vi "MathBuckPr1.vi"() -> ()   [LabVIEW 2015]
uses:
  <vilib>/Simulation/Scripting/Companion Diagram/SimConfigNode/SimParams.ctl
  <vilib>/Simulation/Scripting/Companion Diagram/SimConfigNode/_simSolvers.ctl
  <vilib>/Simulation/Implementation/Shared/SIMSCR Execution Mode.ctl
  <vilib>/Simulation/Param Hierarchy/Typedefs/SIMPH Param Control Actions.ctl
  <vilib>/Simulation/Implementation/Shared/NILVSim_ParamChanged.vi
  <vilib>/Simulation/Implementation/Shared/NILVSIM_BeginStep.vi
  <vilib>/Simulation/Implementation/Shared/NILVSim_Manager.vi
  <vilib>/Utility/error.llb/Clear Errors.vi
  <vilib>/Simulation/Implementation/Shared/NILVSim_FinalizeModel.vi
  <vilib>/imath/engines/lvmath2/RunTimeEngine/Managers/WorkSpace/UID Generator.vi
  <vilib>/imath/engines/lvmath/Plug In/Control Design/BuiltInFunctions/tf/NIMS_CD_tf(STR,Ts).vi
  <vilib>/imathl/engines/lvmath/Functions/Error Handling/Create Error.vi
  <vilib>/imath/engines/lvmath/Plug In/Control Design/BuiltInFunctions/multmx/NIMS_CD_multmx(TF,K).vi
  <vilib>/imath/engines/lvmath/Plug In/Control Design/BuiltInFunctions/powermx/NIMS_CD_powermx(TF,N).vi
  <vilib>/imath/engines/lvmath/Plug In/Control Design/BuiltInFunctions/plus/NIMS_CD_plus(TF,TF).vi
  <vilib>/imath/engines/lvmath/Plug In/Control Design/BuiltInFunctions/plus/NIMS_CD_plus(TF,K).vi
  <vilib>/imath/engines/lvmath/Plug In/Control Design/BuiltInFunctions/multmx/NIMS_CD_multmx(K,TF).vi
  <vilib>/imath/engines/lvmath/Functions/Error Handling/MergeErrorsWrapper.vi
  <vilib>/imath/engines/lvmath/Plug In/Control Design/BuiltInFunctions/plus/NIMS_CD_plus(K,TF).vi
  <vilib>/imath/engines/lvmath/Plug In/Control Design/BuiltInFunctions/rightdivmx/NIMS_CD_rightdivmx(TF,TF).vi
  <vilib>/imath/engines/lvmath/Plug In/Control Design/BuiltInFunctions/rightdivmx/NIMS_CD_rightdivmx(TF,K).vi
  <vilib>/imath/engines/lvmath/Plug In/Control Design/BuiltInFunctions/step/NIMS_CD_[Y,T]=step(TF,[Tinfo]).vi
  <vilib>/imath/engines/lvmath/Plug In/Control Design/BuiltInFunctionSupport/CD_timePlotData(TF).vi
  <vilib>/imath/engines/lvmath/Plug In/Control Design/BuiltInFunctionSupport/Utility_Functions/Plot_Utility/cdmc textMathPlot.vi
  <vilib>/imath/engines/lvmath2/RunTimeEngine/Managers/SymbolTable/Clear UID.vi
  <vilib>/imath/engines/lvmath2/RunTimeEngine/NodeEndStatement/NIMS_NodeEndStatement_Output.vi
  <instcachedir>/0/NIMS_NodeEndStatement_Output_53EC0D466D134D7ABD903AC30B43404B.lvgen/NIMS_NodeEndStatement_Output_53EC0D466D134D7ABD903AC30B43404B_001.vi
  <instcachedir>/0/NIMS_NodeEndStatement_Output_53EC0D466D134D7ABD903AC30B43404B.lvgen/NIMS_NodeEndStatement_Output_53EC0D466D134D7ABD903AC30B43404B_002.vi
  <vilib>/imath/engines/lvmath2/RunTimeEngine/ErrorHandling/NIMS_Finalize Error.vi
  <vilib>/Analysis/Matrix/Numeric/Conversions/Matrix To Array - RM.vi
  <vilib>/Simulation/Implementation/Shared/SIM Unbundle Sim Info.vi
  <vilib>/Simulation/Implementation/Shared/NILVSim_Initialize.vi
  <vilib>/Simulation/Utility/Implementation/NILVSim Get Time and IsAcceptedStep.vi
  <vilib>/Simulation/Implementation/Shared/SIMSH Read Queue.vi
  <vilib>/Simulation/Implementation/Shared/NILVSim_GetModelError.vi
  <vilib>/Simulation/Implementation/Shared/SIM Bundle Sim Info.vi
  <vilib>/Simulation/Scripting/Companion Diagram/SimConfigNode/SimDog.xnode
  <vilib>/Analysis/Matrix/NI_Matrix.lvlib
  <vilib>/Simulation/Implementation/Shared/NI_SIM_Implementation.lvlib
  <vilib>/imath/engines/lvmath2/RunTimeEngine/Managers/SymbolTable/NIMS_WorkSpace.lvlib
panel:
  out "DeltaIL":dbl
  out "P":dbl
  out "Io":dbl
  out "Vo 2":dbl
  in  "error in":errorcluster
  out "Vo":dbl[](graph)
  out "IL":dbl[](graph)
  in  "r":dbl
  in  "D":dbl
  in  "F":dbl
  in  "R":dbl
  in  "C":dbl
  in  "L":dbl
  in  "Vin":dbl
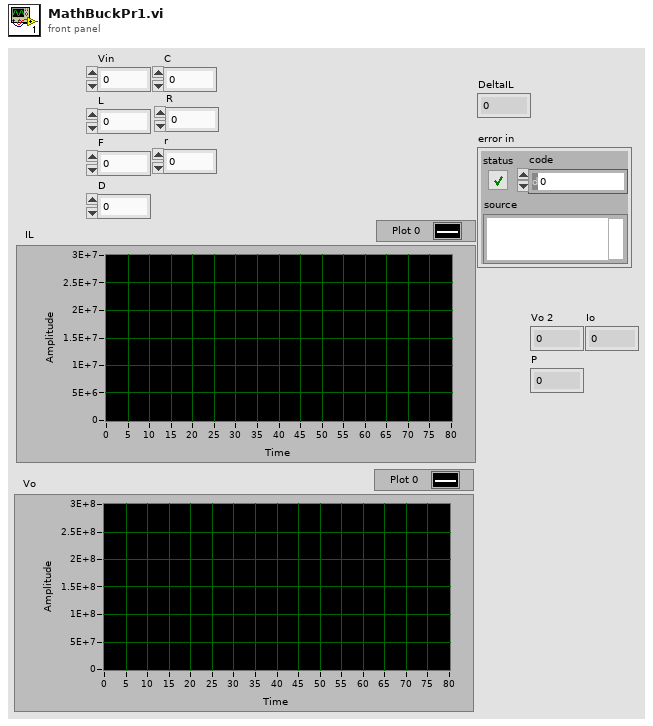
[diagram p1: front panel]
types:
  T1 = cluster{"[0]":i32, "[1]":i32, "[2]":i32, "[3]":i32, "[4]":i32, "[5]":i32, "[6]":i32, "[7]":i32, "[8]":i32}
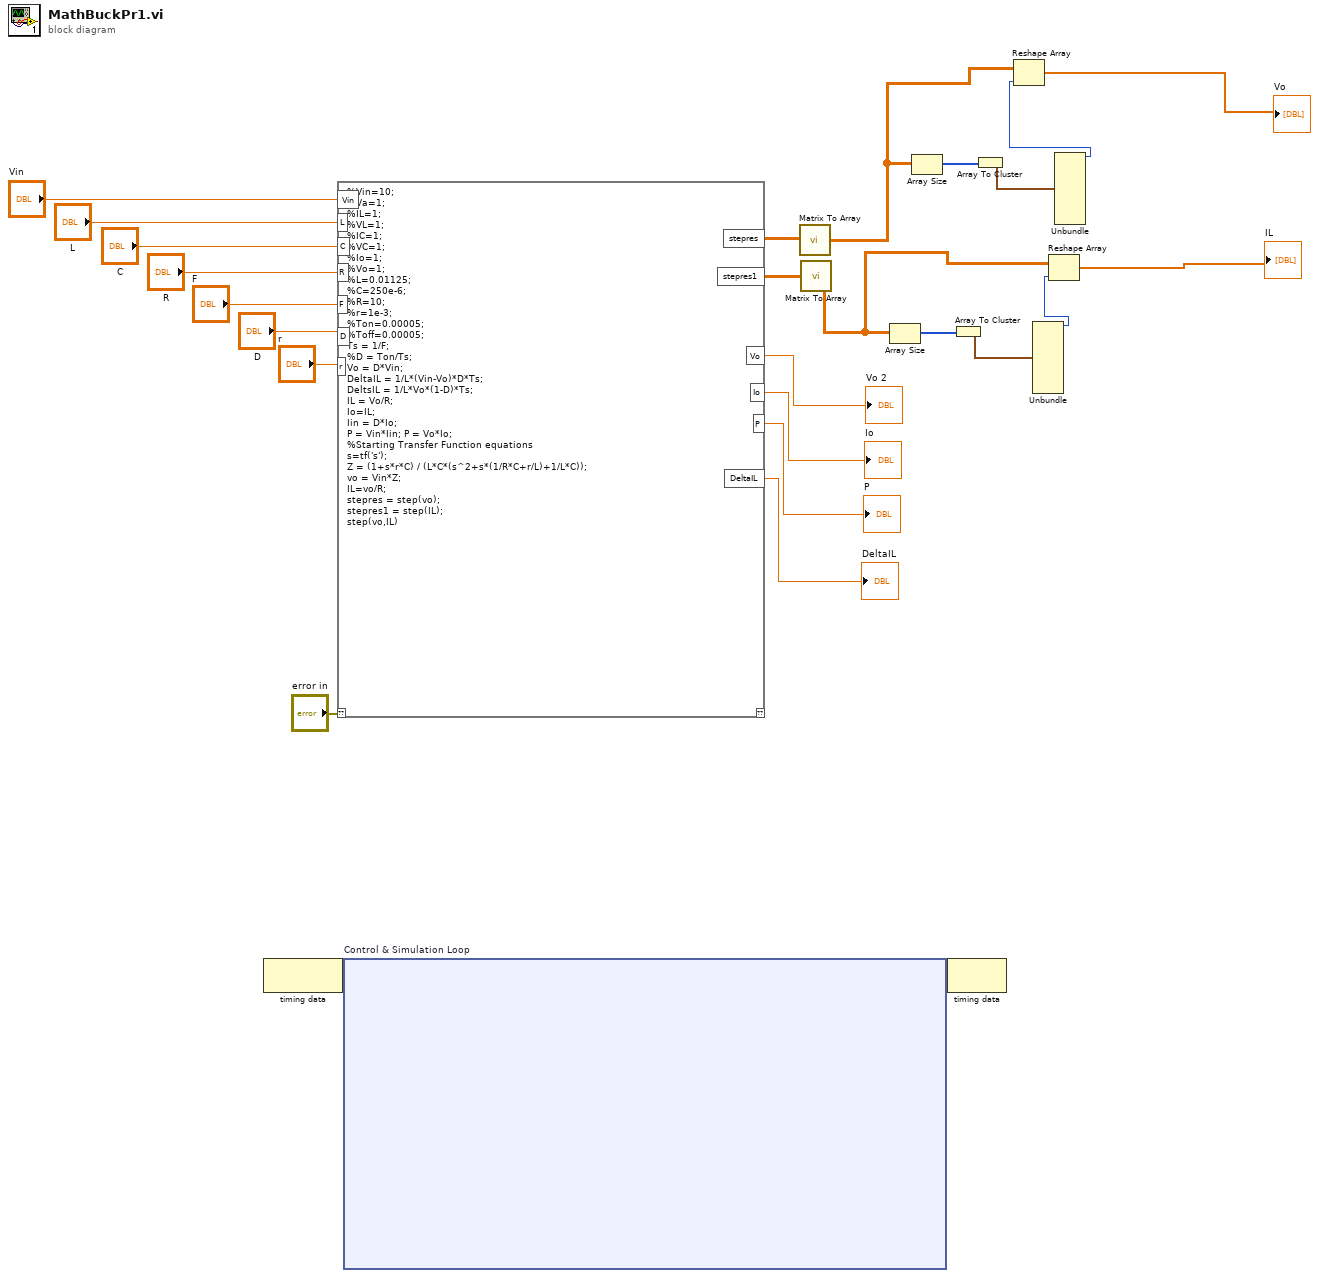
[diagram p0: block diagram]
diagram:
  n1 = node-c288() -> (w2:variant)  [unwired: 1 in]
  n2 = mathscript code="%Vin=10;\n%Va=1;\n%IL=1;\n%VL=1;\n%IC=1;\n%VC=1;\n%Io=1;\n%Vo=1;\n%L=0.01125;\n%C=250e-6;\n%R=10;\n%r=1e-3;\n%Ton=0.00005;\n%Toff=0.00005;\nTs = 1/F;\n%D = Ton/Ts;\nVo = D*Vin;\nDeltaIL = 1/L*(Vin-Vo)*D*Ts;\nDeltsIL = 1/L*Vo*(1-D)*Ts;\nIL = Vo/R;\nIo=IL;\nIin = D*Io;\nP = Vin*Iin; P = Vo*Io;\n%Starting Transfer Function equations\ns=tf('s');\nZ = (1+s*r*C) / (L*C*(s^2+s*(1/R*C+r/L)+1/L*C));\nvo = Vin*Z;\nIL=vo/R;\nstepres = step(vo);\nstepres1 = step(IL);\nstep(vo,IL)"("??"="error in", "Vin"="Vin", "L"="L", "C"="C", "R"="R", "F"="F", "D"="D", "r"="r") -> ("stepres"=w3:dbl[][], "stepres1"=w9:dbl[][], "Vo"=→"Vo 2":dbl, "Io"=→"Io":dbl, "P"=→"P":dbl, "DeltaIL"=→"DeltaIL":dbl)  [unwired: 1 out]
  n3 = node-c254 "Control & Simulation Loop"(w2) -> (w1:variant)
  n4 = call-poly <vilib>:"Matrix To Array.vi"("Real Matrix"=w3) -> ("Real 2D Array"=w14:dbl[][])
  n5 = call-poly <vilib>:"Matrix To Array.vi"("Real Matrix"=w9) -> ("Real 2D Array"=w17:dbl[][])
  n6 = Array Size(array=w17) -> (size(s)=w19:i32[])
  n7 = Array Size(array=w14) -> (size(s)=w16:i32[])
  n8 = node-c288(w1) -> ()  [unwired: 1 out]
  n9 = Array To Cluster(array=w19) -> (cluster=w18:T1)
  n10 = Array To Cluster(array=w16) -> (cluster=w15:T1)
  n11 = Unbundle(w18) -> ("[0]"=w13:i32)  [unwired: 8 out]
  n12 = Reshape Array(w17, w13) -> (→"IL":dbl[])
  n13 = Unbundle(w15) -> ("[0]"=w12:i32)  [unwired: 8 out]
  n14 = Reshape Array(w14, w12) -> (→"Vo":dbl[])
